vi "initialize_lib_tsmaster_win32.vi"(0 "初始化CAN通道":T1 {"LIN使用通道数" max=5; "CAN使用通道数" max=5}, 11 "错误输入（无错误）":errorcluster) -> (4 "initialize_lib_tsmaster":i32, 6 "应用程序名":string, 8 "InitializationInformation":T1 {"LIN使用通道数" max=5; "CAN使用通道数" max=5}, 15 "错误输出":errorcluster)   [LabVIEW 2016]
uses:
  Ctrl/CAN_Info.ctl
  TSMaster.dll
panel:
  out "initialize_lib_tsmaster_ok":bool
  # "用于配置参数->应用程序名所指定代码所使用的CAN的通道数和lin的通道数\n返回值用于判断是否成功，\n返回值：\ninitialize_lib_tsmaster->函数错误代码，0为正常，其他请参阅故障码表，后续会加上"
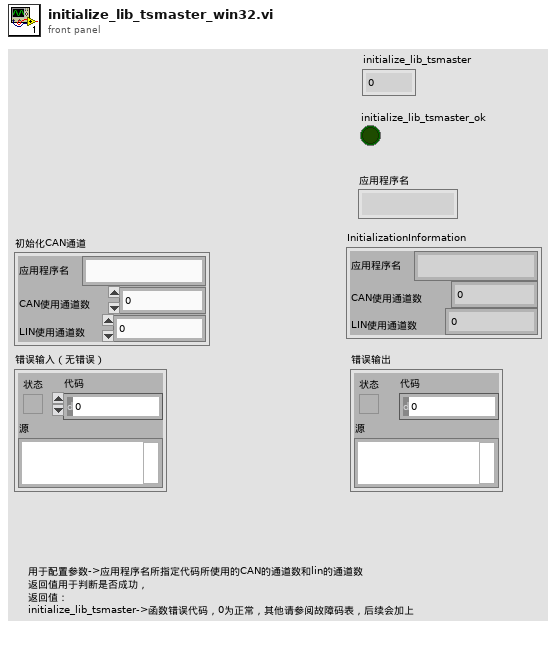
[diagram p1: front panel]
types:
  T1 = typedef "CAN_Info.ctl" = cluster{"应用程序名":string, "CAN使用通道数":u8, "LIN使用通道数":u8}
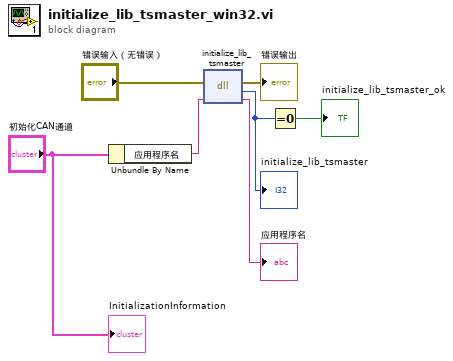
[diagram p0: block diagram]
diagram:
  n1 = Unbundle By Name("初始化CAN通道") -> ("应用程序名"=w7:string)
  n2 = dll-call lib="C:/Users/Eric/Desktop/LabVIEW/TSMasterAPI/Win32/CANopen_TS_2015/TSMaster.dll" fn="initialize_lib_tsmaster"(error in="错误输入（无错误）", "AAppName"=w7) -> (error out=→"错误输出":errorcluster, "initialize_lib_tsmaster"=w3:i32, "AAppName"=→"应用程序名":string)  [unwired: 2 in, 1 out]
  "initialize_lib_tsmaster" <- w3
  n3 = Equal To 0?(x=w3) -> (x = 0?=→"initialize_lib_tsmaster_ok":bool)
  "InitializationInformation" <- "初始化CAN通道"
